vi "Init.vi"(8 "error in (no error)":errorcluster, 11 "Port In":refnum<visa-resource-name>="COM14") -> (0 "error out":errorcluster, 2 "Model (9625)":u32, 3 "Port Out":refnum<visa-resource-name>="COM14")   [LabVIEW 2023, in "Temperature Controller.lvlib"]
uses:
  <vilib>/Instr/_visa.llb/VISA Configure Serial Port (Instr).vi
  Temperature Controller.lvlib
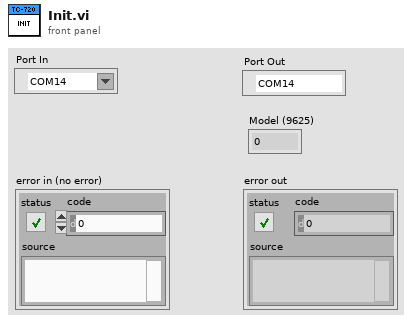
[diagram p1: front panel]
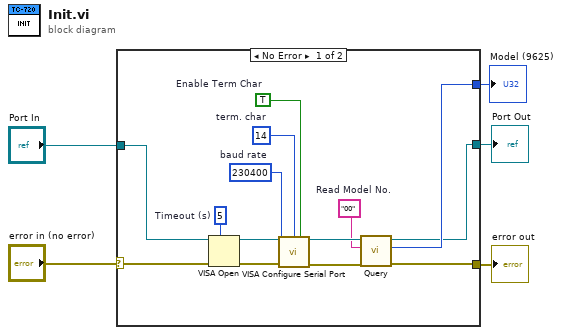
[diagram p0: block diagram]
diagram:
  n1 = case shown="No Error" "error in (no error)" {
    selector: "error in (no error)" -> [w12 w20]
    tunnel: "Port In" -> [w15 w21]
    tunnel: [w6 w21] -> w4
    tunnel: [w8 w20] -> w3
    tunnel: [w7 _] -> w1
    frame No Error {
      w9 = "00"  # Read Model No.
      w13 = TRUE  # Enable Term Char
      w16 = u8 14  # term. char
      w17 = u32 230400  # baud rate
      w19 = u32 5  # Timeout (s)
      n2 = VISA Open(timeout (0)=w19, error in (no error)=w12, VISA resource name=w15) -> (VISA resource name=w18:refnum<visa-resource-name>, error out=w14:errorcluster)  [unwired: 1 in, 1 out]
      n3 = call-poly "VISA Configure Serial Port"("VISA resource name"=w18, "termination char\n(0xA = '\\n' = LF)"=w16, "Enable Termination\nChar (T)"=w13, "baud rate (9600)"=w17, "error in (no error)"=w14) -> ("VISA resource name out"=w10:refnum<visa-resource-name>, "error out"=w11:errorcluster)  [unwired: 9 in]
      n4 = call "Query.vi"("error in (no error)"=w11, "Command"=w9, "Port In"=w10) -> ("error out"=w8:errorcluster, "Reply Int"=w7:u32, "Port Out"=w6:refnum<visa-resource-name>)  [unwired: 4 in, 2 out]
    }
    frame Error {
    }
  }
  "Port Out" <- w4
  "error out" <- w3
  "Model (9625)" <- w1
